vi "ScanAction.vi"(8 "error in (no error)":errorcluster caption="entrée d'erreur (pas d'erreur)", 9 "IndicePoint":i32, 10 "Dir":bool, 11 "Tools In":refnum<class "AndorSpectro.lvclass"> caption="DNL_LabVIEW Object in") -> (0 "error out":errorcluster caption="sortie d'erreur", 2 "ScanParsOut":dbl[](array[numeric]), 3 "Tools Out":refnum<class "AndorSpectro.lvclass"> caption="DNL_LabVIEW Object out")   [LabVIEW 2019, in "AndorSpectro.lvclass"]
uses:
  AndorSpectro.lvclass
  C:/Programmes Labview/LabscanV1A/DevicesClass/BaseDevice/BaseDevice.lvclass
  AndorSpectro.lvclass/AndorSpectro.ctl
  <userlib>/ATSpectrograph/atspectrograph.lvlib
panel:
  in  "CamUpdate":bool
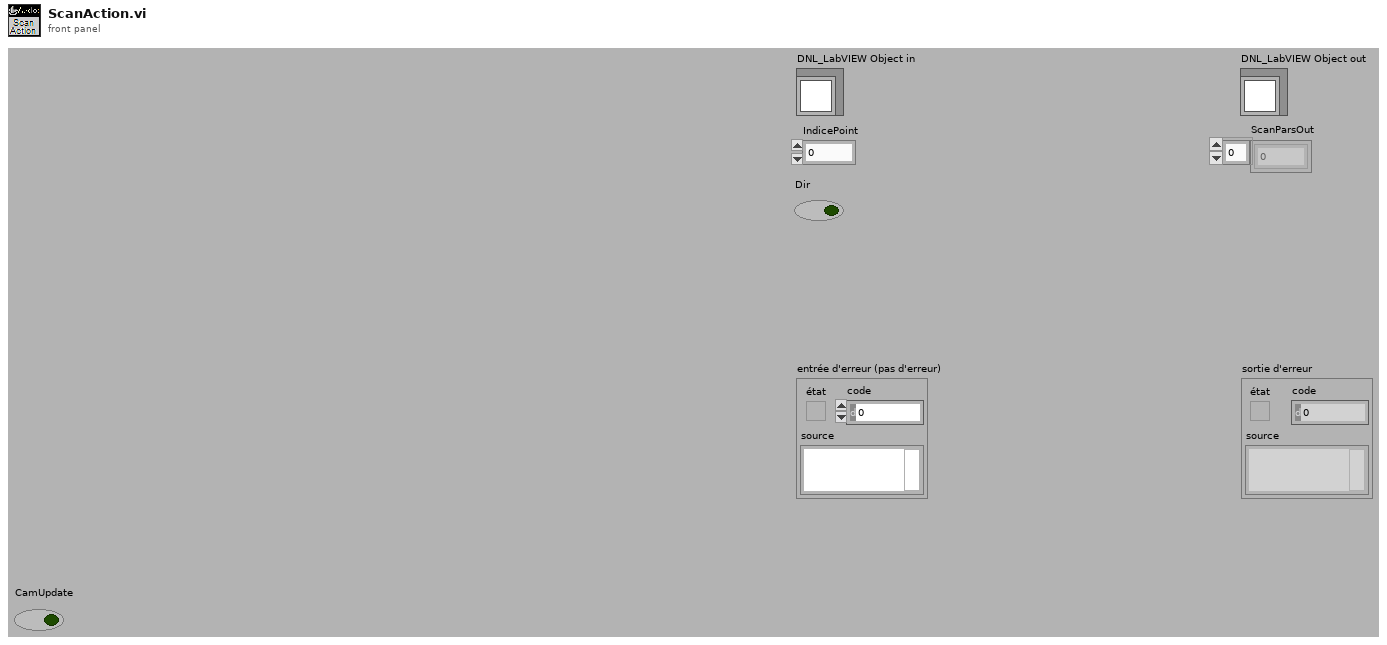
[diagram p1: front panel]
types:
  T1 = typedef "AndorSpectro.lvclass/AndorSpectro_Func.ctl" = enum16{"ReadSpectrum (cnt)", "SetWavelenght (nm)"}
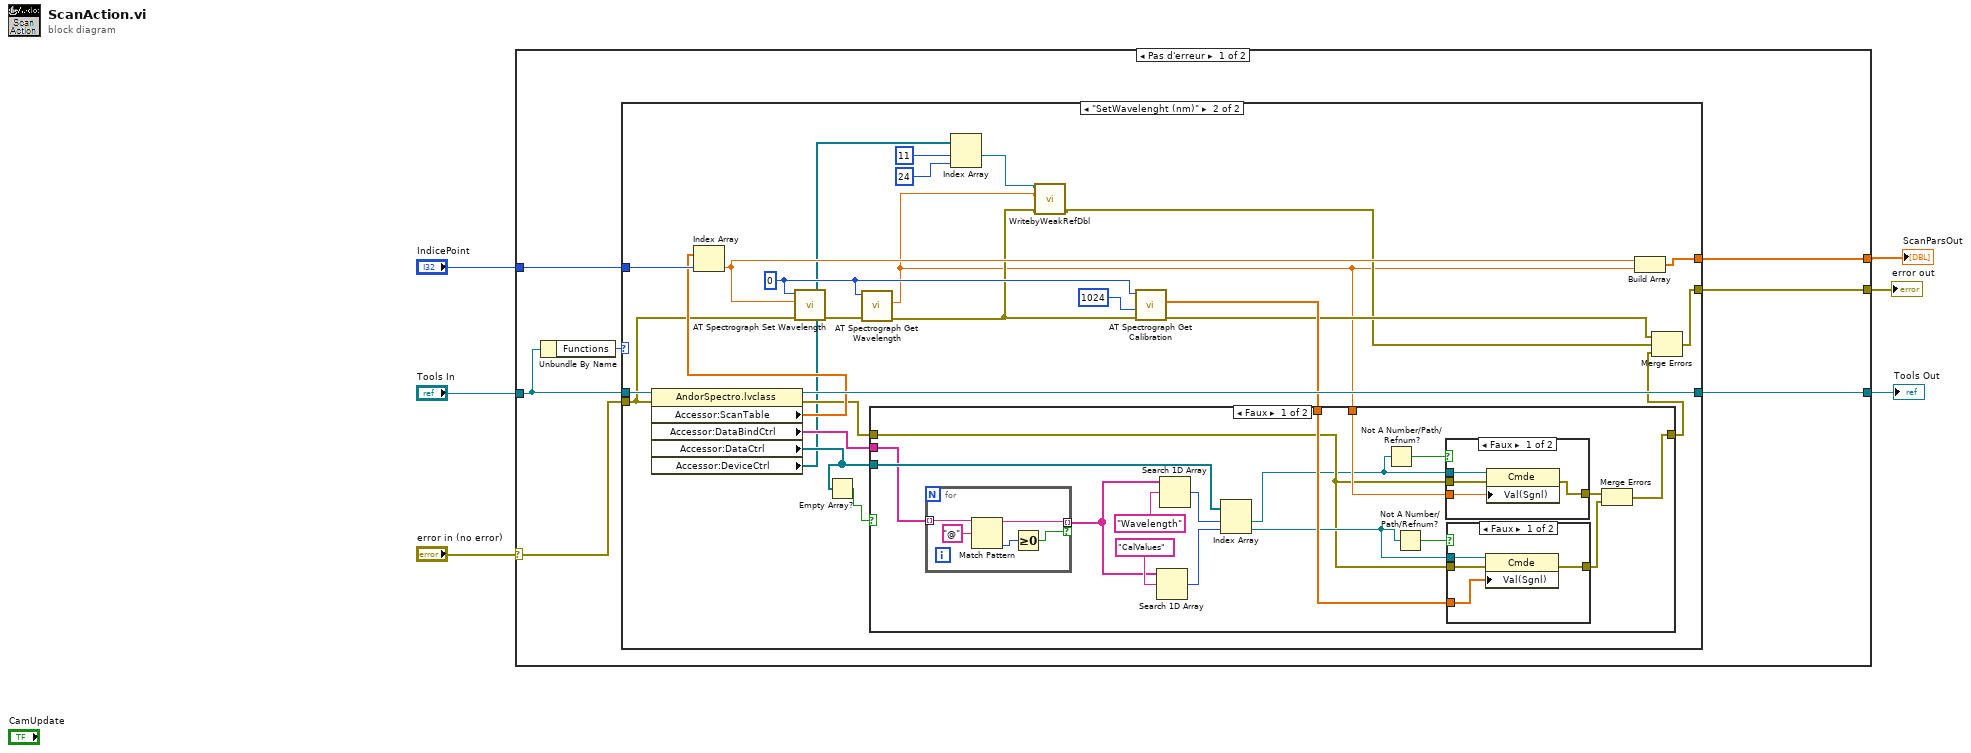
[diagram p0: block diagram]
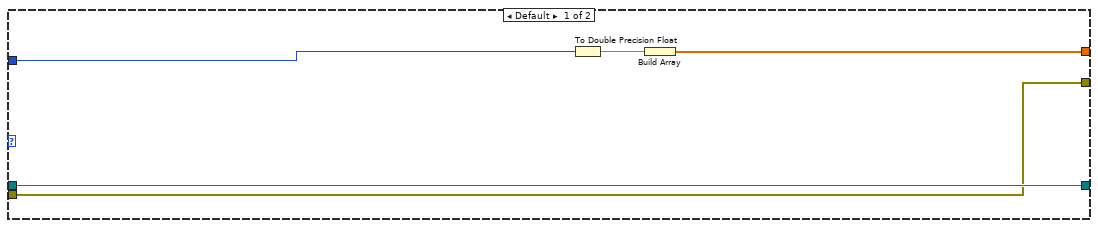
[diagram p2: hidden frame]
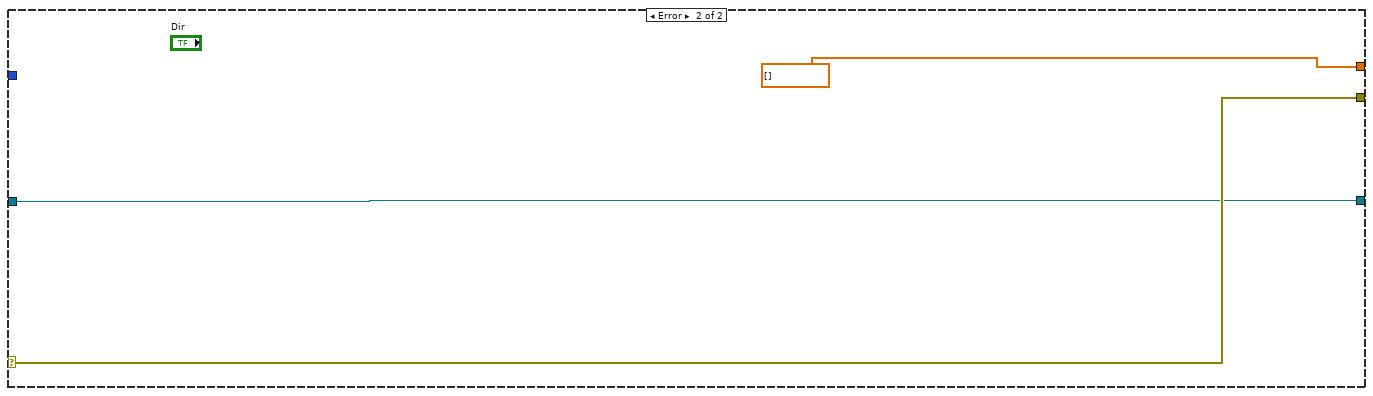
[diagram p6: hidden frame]
diagram:
  n1 = case shown="Pas d'erreur" "error in (no error)" {
    selector: "error in (no error)" -> [w10 w79]
    tunnel: "Tools In" -> [w11 w78]
    tunnel: [w9 dbl[] []] -> w1
    tunnel: [w8 w79] -> w4
    tunnel: [w7 w78] -> w3
    tunnel: "IndicePoint" -> [w12 _]
    frame No Error {
      n2 = Unbundle By Name(w11) -> ("Functions"=w13:T1)
      n3 = case shown="\"SetWavelenght (nm)\"" w13 {
        tunnel: [w14 w35] -> w9
        tunnel: w12 -> [w18 w38]
        tunnel: [w16 w39] -> w7
        tunnel: w11 -> [w16 w40]
        tunnel: w10 -> [w15 w30]
        tunnel: [w15 w27] -> w8
        frame Default {
          n4 = To Double Precision Float(number=w18) -> (double precision float=w17:dbl)
          n5 = Build Array(w17) -> (w14:dbl[])
        }
        frame "SetWavelenght (nm)" {
          w41 = 0 ("device")
          n6 = property class="AndorSpectro.lvclass"(reference=w40, error in=w30) -> (reference out=w39:refnum<class "AndorSpectro.lvclass">, error out=w31:errorcluster, "Accessor:ScanTable"=w37:dbl[], "Accessor:DataBindCtrl"=w33:string[], "Accessor:DataCtrl"=w32:refnum<vi>[], "Accessor:DeviceCtrl"=w23:refnum<vi>[])
          n7 = Index Array(array=w37, index=w38) -> (element=w36:dbl)
          n8 = call <userlib>:"AT Spectrograph Set Wavelength.vi"("error in (no error)"=w30, "wavelength"=w36, "device"=w41) -> ("error out"=w42:errorcluster)  [unwired: 7 in, 1 out]
          n9 = Empty Array?(array=w32) -> (empty?=w34:bool)
          n10 = call <userlib>:"AT Spectrograph Get Wavelength.vi"("error in (no error)"=w42, "device"=w41) -> ("error out"=w21:errorcluster, "wavelength out"=w20:sgl)  [unwired: 7 in, 1 out]
          n11 = Index Array(array=w23, index #1=11 ("indice"), index #2=24 ("indice")) -> (element #1=w19:refnum<vi>)  [unwired: 1 out]
          n12 = call <userlib>:"WritebyWeakRefDbl.vi"("error in"=w21, "Valeur"=w20, "Control Ref"=w19) -> ("error out"=w22:errorcluster)  [unwired: 8 in]
          n13 = call <userlib>:"AT Spectrograph Get Calibration.vi"("error in (no error)"=w21, "numberPixels"=1024, "device"=w41) -> ("error out"=w28:errorcluster, "calibrationValuesOut"=w29:sgl[])  [unwired: 5 in, 1 out]
          n14 = case shown="Faux" w34 {
            tunnel: w33 -> [w55 _]
            tunnel: w32 -> [w56 _]
            tunnel: w31 -> [w46 w76]
            tunnel: [w44 w76] -> w26
            tunnel: w20 -> [w49 _]
            tunnel: w29 -> [w48 _]
            frame False {
              n15 = for {
                tunnel: w55 -> [w75] mode=indexing
                tunnel: [w73] -> w54 mode=indexing if=w72
                n16 = Match Pattern(string=w75, regular expression="@" ("expression régulière")) -> (before substring=w73:string, offset past match=w71:i32)  [unwired: 1 in, 2 out]
                n17 = Greater Or Equal To 0?(x=w71) -> (x >= 0?=w72:bool)
              }
              n18 = Search 1D Array(1D array=w54, element="CalValues" ("nom (aucun)")) -> (index of element=w57:i32)  [unwired: 1 in]
              n19 = Search 1D Array(1D array=w54, element="Wavelength" ("nom (aucun)")) -> (index of element=w59:i32)  [unwired: 1 in]
              n20 = Index Array(array=w56, index #1=w59, index #2=w57) -> (element #1=w45:refnum<vi>, element #2=w47:refnum<vi>)
              n21 = Not A Number/Path/Refnum?(number/path/refnum=w45) -> (NaN/Path/Refnum?=w50:bool)
              n22 = Not A Number/Path/Refnum?(number/path/refnum=w47) -> (NaN/Path/Refnum?=w51:bool)
              n23 = case shown="Faux" w50 {
                tunnel: w45 -> [w69 _]
                tunnel: w49 -> [w68 _]
                tunnel: w46 -> [w67 w70]
                tunnel: [w66 w70] -> w52
                frame False {
                  n24 = property class="Cmde"(reference=w69, error in=w67, "Val(Sgnl)"=w68) -> (error out=w66:errorcluster)  [unwired: 1 out]
                }
                frame True {
                }
              }
              n25 = case shown="Faux" w51 {
                tunnel: w47 -> [w64 _]
                tunnel: w46 -> [w61 w65]
                tunnel: [w63 w65] -> w53
                tunnel: w48 -> [w62 _]
                frame False {
                  n26 = property class="Cmde"(reference=w64, error in=w61, "Val(Sgnl)"=w62) -> (error out=w63:errorcluster)  [unwired: 1 out]
                }
                frame True {
                }
              }
              n27 = Merge Errors(w52, w53) -> (w44:errorcluster)
            }
            frame True {
            }
          }
          n28 = Build Array(w36, w20) -> (w35:dbl[])
          n29 = Merge Errors(w28, w22, w26) -> (w27:errorcluster)
        }
      }
    }
    frame Error {
    }
  }
  "error out" <- w4
  "Tools Out" <- w3
  "ScanParsOut" <- w1
